vi "Building_Origin_of_Tracks(101)-1.vi"(4 "[IN] # part of \norigin track":i32, 5 "error IN":errorcluster, 6 "[IN] Subtrack":T1, 7 "[IN] Problem point \nin the origin":i32, 8 "[IN] Still connected\ntracks in group":T2) -> (0 "error OUT":errorcluster, 1 "[OUT] Subtrack":T1, 2 "[OUT] Last point in subtrack":i32)   [LabVIEW 2013]
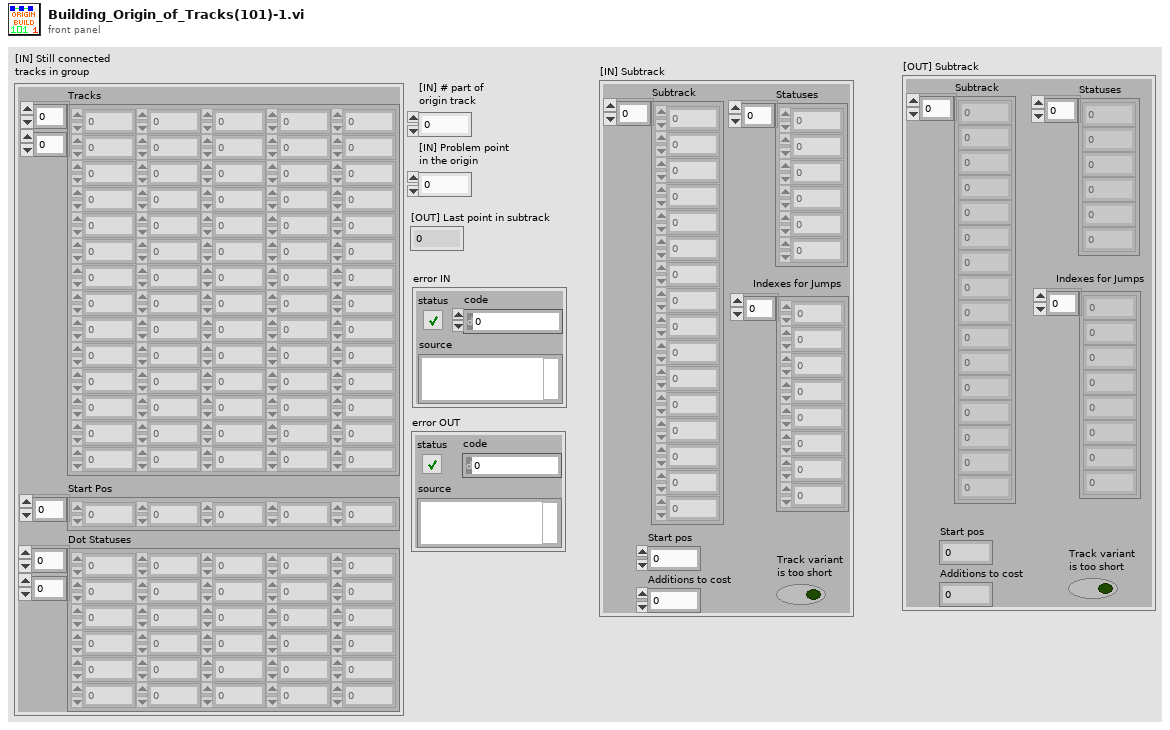
[diagram p1: front panel]
types:
  T1 = cluster{"Subtrack":dbl[], "Statuses":i16[], "Start pos":i32, "Additions to cost":i32, "Track variant \nis too short":bool, "Indexes for Jumps":i32[]}
  T2 = cluster{"Tracks":dbl[][], "Start Pos":i32[], "Dot Statuses":i16[][]}
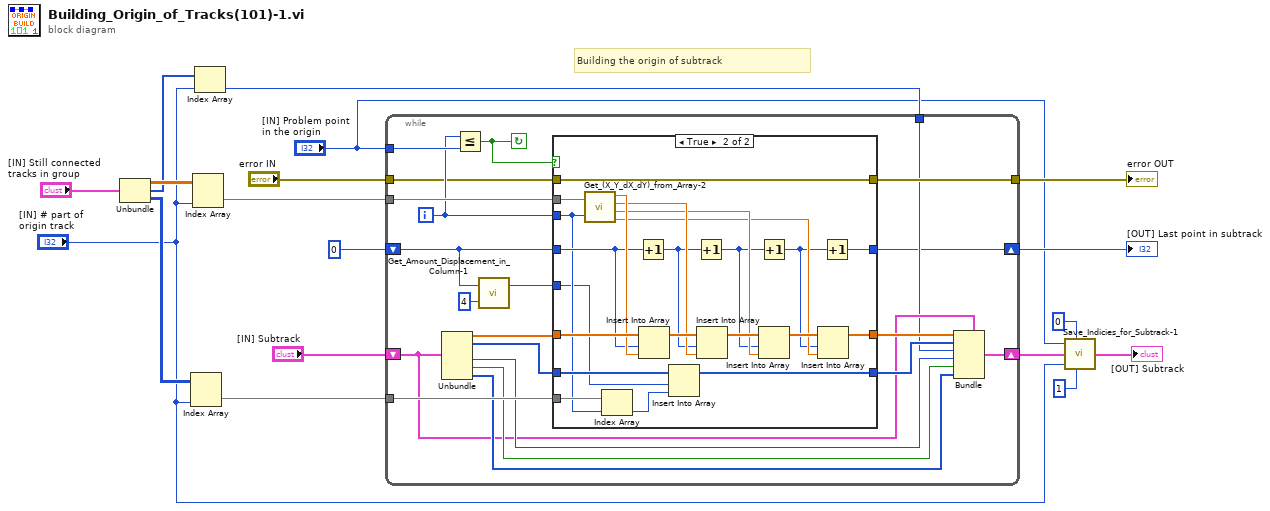
[diagram p0: block diagram]
diagram:
  # "Building the origin of subtrack"
  n1 = Unbundle("[IN] Still connected\ntracks in group") -> ("Tracks"=w15:dbl[][], "Start Pos"=w13:i32[], "Dot Statuses"=w11:i16[][])
  n2 = Index Array(array=w11, index (col)="[IN] # part of \norigin track") -> (element=w10:i16[])  [unwired: 1 in]
  n3 = Index Array(array=w15, index (col)="[IN] # part of \norigin track") -> (element=w14:dbl[])  [unwired: 1 in]
  n4 = Index Array(array=w13, index="[IN] # part of \norigin track") -> (element=w12:i32)
  n5 = while {
    tunnel: w14 -> [w39]
    tunnel: w10 -> [w35]
    shift-right: [w30] -> w6
    shift-left: "[IN] Subtrack" -> [w24]
    tunnel: "[IN] Problem point \nin the origin" -> [w34]
    tunnel: "error IN" -> [w26]
    tunnel: [w25] -> w8
    tunnel: w12 -> [w23]
    shift-right: [w22] -> w9
    shift-left: 0 -> [w20]
    i -> [w33]
    stop <- w37 continue-if-true
    n6 = Unbundle(w24) -> ("Subtrack"=w38:dbl[], "Statuses"=w36:i16[], "Additions to cost"=w29:i32, "Track variant \nis too short"=w28:bool, "Indexes for Jumps"=w27:i32[])  [unwired: 1 out]
    n7 = Less Or Equal?(x=w33, y=w34) -> (x <= y?=w37:bool)
    n8 = call "Get_Amount_Displacement_in_Column-1.vi"("multiplier"=4, "# Rows"=w20) -> ("Displ amount"=w19:i32)  [unwired: 1 out]
    n9 = case shown="True" w37 {
      tunnel: w39 -> [_ w65]
      tunnel: w38 -> [w42 w64]
      tunnel: w20 -> [w40 w62]
      tunnel: w33 -> [_ w51]
      tunnel: w36 -> [w43 w53]
      tunnel: w35 -> [_ w52]
      tunnel: [w42 w49] -> w32
      tunnel: [w43 w48] -> w31
      tunnel: w26 -> [w41 w47]
      tunnel: [w41 w47] -> w25
      tunnel: [w40 w44] -> w22
      tunnel: w19 -> [_ w46]
      frame False {
      }
      frame True {
        n10 = call "Get_(X_Y_dX_dY)_from_Array-2.vi"("(X,Y,dX,dY)"=w65, "Index of Displacement"=w51) -> ("X"=w63:dbl, "Y"=w60:dbl, "dX"=w57:dbl, "dY"=w54:dbl)
        n11 = Index Array(array=w52, index=w51) -> (element=w50:i16)
        n12 = Increment(x=w62) -> (x+1=w58:i32)
        n13 = Insert Into Array(array=w64, index=w62, new element=w63) -> (w61:dbl[])
        n14 = Insert Into Array(array=w53, index=w46, new element=w50) -> (w48:i16[])
        n15 = Increment(x=w58) -> (x+1=w56:i32)
        n16 = Insert Into Array(array=w61, index=w58, new element=w60) -> (w59:dbl[])
        n17 = Increment(x=w56) -> (x+1=w45:i32)
        n18 = Insert Into Array(array=w59, index=w56, new element=w57) -> (w55:dbl[])
        n19 = Insert Into Array(array=w55, index=w45, new element=w54) -> (w49:dbl[])
        n20 = Increment(x=w45) -> (x+1=w44:i32)
      }
    }
    n21 = Bundle(cluster=w24, "Subtrack"=w32, "Statuses"=w31, "Start pos"=w23, "Additions to cost"=w29, "Track variant \nis too short"=w28, "Indexes for Jumps"=w27) -> (w30:T1)
  }
  "[OUT] Last point in subtrack" <- w9
  "error OUT" <- w8
  n22 = call "Save_Indicies_for_Subtrack-1.vi"("[IN] Index of Origin/Problem \nPoint inside Original Track (X1)"="[IN] Problem point \nin the origin", "[IN] i for X1"=0, "[IN] Subtrack"=w6, "[IN] Index of Track Conta-\nining Origin/Problem (X2)"="[IN] # part of \norigin track", "[IN] i for X2"=1 ("[IN] i for X1")) -> ("[OUT] Subtrack"=→"[OUT] Subtrack":T1)
